vi "IT-M7700 Application waveform output.vi"() -> ()   [LabVIEW 2015]
doc: "This example is used to edit the parameters of the application waveform, output the waveform, and display the voltage and current read-back values in real time."
uses:
  <instrlib>/IT-M7700/IT-M7700.lvlib
panel:
  in  "OCP Delay(ms)":i32 min=0 max=9999
  in  "RMS OCP Level(A)":dbl min=0.0 format="%.2g"
  in  "Wave":u16(ring) items=["SINE", "SQUA", "TRIANGLE", "SAW", "CLIPSINE"]
  in  "Stop Phase(°)":dbl min=0.0 format="%.2g"
  in  "Start Phase(°)":dbl min=0.0 format="%.2g"
  in  "Frequency(HZ)":dbl min=0.0 format="%.2g"
  in  "AC Level(V)":dbl min=0.0 format="%.2g"
  in  "Serial Configuration":T1={"Baud Rate"=9600, "Parity"=0, "Data Bits"=8, "Stop Bits"=10, "Flow Control"=0} {"Flow Control" items=["None", "XON/XOFF", "RTS/CTS", "XON/XOFF & RTS/CTS", "DTR/DSR", "XON/XOFF & DTR/DSR"]; "Stop Bits" items=["1.0"=10, "1.5"=15, "2.0"=20]; "Data Bits" items=["7"=7, "8"=8]; "Parity" items=["None", "Odd", "Even", "Mark", "Space"]; "Baud Rate" items=["1200"=1200, "2400"=2400, "4800"=4800, "9600"=9600, "19200"=19200, "34800"=34800, "57600"=57600, "115200"=115200]}
  in  "VISA resource name":refnum<visa-resource-name>
  out "Read AC Voltage(V)":dbl format="%.3g"
  out "Read AC Current(A)":dbl format="%.3g"
  out "Read Power(W)":dbl format="%.3g"
  in  "?":bool
  # "Application Wave Output"
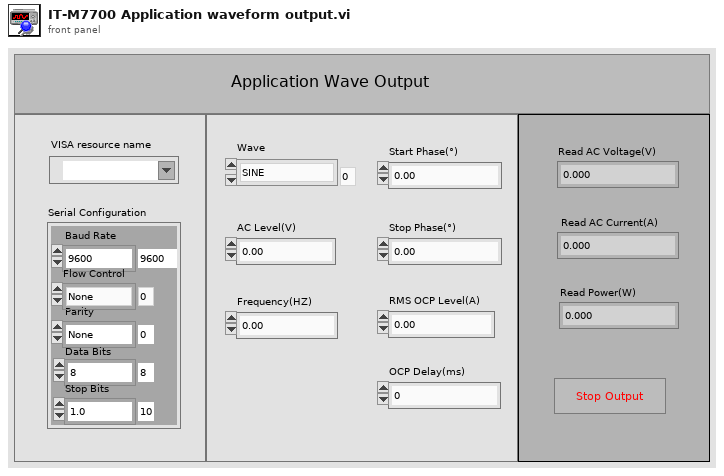
[diagram p1: front panel]
types:
  T1 = cluster{"Baud Rate":u32, "Parity":u16, "Data Bits":u16, "Stop Bits":u16, "Flow Control":u16}
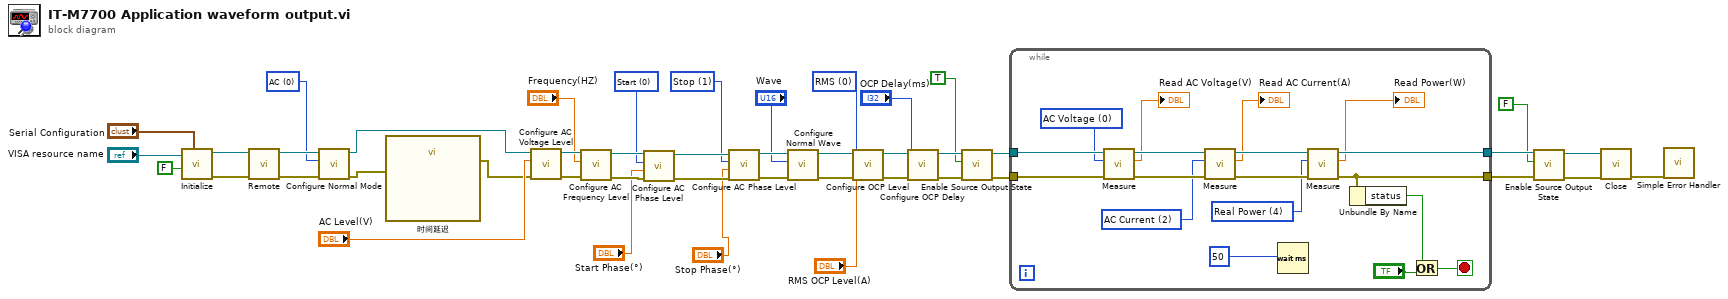
[diagram p0: block diagram]
diagram:
  w38 = u16 0 items=["RMS", "PEAK"] ("Type")
  w13 = u16 1 items=["Start", "Stop"] ("Type")
  w14 = u16 0 items=["Start", "Stop"] ("Type")
  w23 = u16 0 items=["AC", "DC", "AC+DC"] ("Mode")
  n1 = call <instrlib>:"Initialize.vi"("Serial Configuration"="Serial Configuration", "Reset"=FALSE, "VISA resource name"="VISA resource name") -> ("error out"=w42:errorcluster, "VISA resource name out"=w43:refnum<visa-resource-name>)  [unwired: 7 in]
  n2 = call <instrlib>:"Remote.vi"("error in"=w42, "VISA resource name"=w43) -> ("error out"=w24:errorcluster, "VISA resource name out"=w25:refnum<visa-resource-name>)  [unwired: 8 in]
  n3 = call <instrlib>:"Configure Normal Mode.vi"("error in"=w24, "Mode"=w23, "VISA resource name"=w25) -> ("error out"=w3:errorcluster, "VISA resource name out"=w4:refnum<visa-resource-name>)  [unwired: 7 in]
  n4 = call "时间延迟"("error in (no error)"=w3) -> ("error out"=w2:errorcluster)  [unwired: 10 in]
  n5 = call <instrlib>:"Configure AC Voltage Level.vi"("error in"=w2, "Level(V)"="AC Level(V)", "VISA resource name"=w4) -> ("error out"=w21:errorcluster, "VISA resource name out"=w22:refnum<visa-resource-name>)  [unwired: 7 in]
  n6 = call <instrlib>:"Configure AC Frequency Level.vi"("error in"=w21, "Frequency(HZ)"="Frequency(HZ)", "VISA resource name"=w22) -> ("error out"=w17:errorcluster, "VISA resource name out"=w18:refnum<visa-resource-name>)  [unwired: 7 in]
  n7 = call <instrlib>:"Configure AC Phase Level.vi"("error in"=w17, "Phase(°)"="Start Phase(°)", "Type"=w14, "VISA resource name"=w18) -> ("error out"=w15:errorcluster, "VISA resource name out"=w16:refnum<visa-resource-name>)  [unwired: 6 in]
  n8 = call <instrlib>:"Configure AC Phase Level.vi"("error in"=w15, "Phase(°)"="Stop Phase(°)", "Type"=w13, "VISA resource name"=w16) -> ("error out"=w9:errorcluster, "VISA resource name out"=w10:refnum<visa-resource-name>)  [unwired: 6 in]
  n9 = call <instrlib>:"Configure Normal Wave.vi"("error in"=w9, "Wave"="Wave", "VISA resource name"=w10) -> ("error out"=w7:errorcluster, "VISA resource name out"=w8:refnum<visa-resource-name>)  [unwired: 7 in]
  n10 = call <instrlib>:"Configure OCP Level.vi"("error in"=w7, "Level(A)"="RMS OCP Level(A)", "Type"=w38, "VISA resource name"=w8) -> ("error out"=w39:errorcluster, "VISA resource name out"=w40:refnum<visa-resource-name>)  [unwired: 6 in]
  n11 = call <instrlib>:"Configure OCP Delay.vi"("error in"=w39, "Delay(ms)"="OCP Delay(ms)", "VISA resource name"=w40) -> ("error out"=w29:errorcluster, "VISA resource name out"=w30:refnum<visa-resource-name>)  [unwired: 7 in]
  n12 = call <instrlib>:"Enable Source Output State.vi"("error in"=w29, "State"=TRUE, "VISA resource name"=w30) -> ("error out"=w27:errorcluster, "VISA resource name out"=w28:refnum<visa-resource-name>)  [unwired: 7 in]
  n13 = while {
    tunnel: w28 -> [w62]
    tunnel: w27 -> [w61]
    tunnel: [w56] -> w34
    tunnel: [w46] -> w35
    stop <- w47 stop-if-true
    w49 = u16 4 items=["AC Voltage", "DC Voltage", "AC Current", "DC Current", "Real Power", "Apparent Power", "Pfactor Power", "Frequency", "THD", "Current THD", "Reactive Power"] ("Measure Type")
    w50 = u16 2 items=["AC Voltage", "DC Voltage", "AC Current", "DC Current", "Real Power", "Apparent Power", "Pfactor Power", "Frequency", "THD", "Current THD", "Reactive Power"] ("Measure Type")
    w51 = u16 0 items=["AC Voltage", "DC Voltage", "AC Current", "DC Current", "Real Power", "Apparent Power", "Pfactor Power", "Frequency", "THD", "Current THD", "Reactive Power"] ("Measure Type")
    n14 = call <instrlib>:"Measure.vi"("error in"=w61, "Measure Type"=w51, "VISA resource name"=w62) -> ("error out"=w59:errorcluster, "Measurement"=→"Read AC Voltage(V)":dbl, "VISA resource name out"=w60:refnum<visa-resource-name>)  [unwired: 6 in]
    n15 = call <instrlib>:"Measure.vi"("error in"=w59, "Measure Type"=w50, "VISA resource name"=w60) -> ("error out"=w57:errorcluster, "Measurement"=→"Read AC Current(A)":dbl, "VISA resource name out"=w58:refnum<visa-resource-name>)  [unwired: 6 in]
    n16 = Wait (ms)(milliseconds to wait=50) -> ()  [unwired: 1 out]
    n17 = call <instrlib>:"Measure.vi"("error in"=w57, "Measure Type"=w49, "VISA resource name"=w58) -> ("error out"=w46:errorcluster, "Measurement"=→"Read Power(W)":dbl, "VISA resource name out"=w56:refnum<visa-resource-name>)  [unwired: 6 in]
    n18 = Unbundle By Name(w46) -> ("status"=w45:bool)
    n19 = Or(x=w45, y="?") -> (x .or. y?=w47:bool)
  }
  n20 = call <instrlib>:"Enable Source Output State.vi"("error in"=w35, "State"=FALSE, "VISA resource name"=w34) -> ("error out"=w32:errorcluster, "VISA resource name out"=w33:refnum<visa-resource-name>)  [unwired: 7 in]
  n21 = call <instrlib>:"Close.vi"("error in"=w32, "VISA resource name"=w33) -> ("error out"=w41:errorcluster)  [unwired: 9 in]
  n22 = call <vilib>:"Simple Error Handler.vi"("error in (no error)"=w41) -> ()  [unwired: 4 in, 5 out]
